vi "interface_configuration.vi"(8 "error in (no error)":errorcluster, 11 "config in":T1) -> (0 "error out":errorcluster, 3 "config out":T1)   [LabVIEW 2015, in "lv-builder-default.lvlib"]
uses:
  lv-builder-default.lvlib
  _controls/post_action_lvlib.ctl
  _controls/post_action_installer.ctl
  _controls/post_action_application.ctl
  _controls/post_action_zip.ctl
  community/_controls/configuration.ctl
  <vilib>/Utility/error.llb/Error Cluster From Error Code.vi
  <vilib>/ErrorRing/Error Ring.xnode
panel:
  in  "distribution_folder":path caption="Distribution Folder"
  in  "dependencies_folder":path caption="Dependencies Folder"
  in  "bin_folder":path caption="Bin Path"
  in  "application_post_action":T2 caption="Application Post Action"
  in  "cancel":bool
  in  "save":bool
  in  "installer_post_file":path caption="Installer Post File"
  in  "zip_move_directory":path caption="Archive Directory"
  in  "zip_post_action":T3 caption="Archive Post Action"
  in  "installer_post_action":T4 caption="Installer Post Action"
  in  "update_version_vi":path caption="Update Version VI"
  in  "lvlibp_move_directory":path caption="lvlibp Directory"
  in  "lvlib_move_directory":path caption="lvlib Directory"
  in  "lvlib_post_action":T5 caption="LVLIB Post Action"
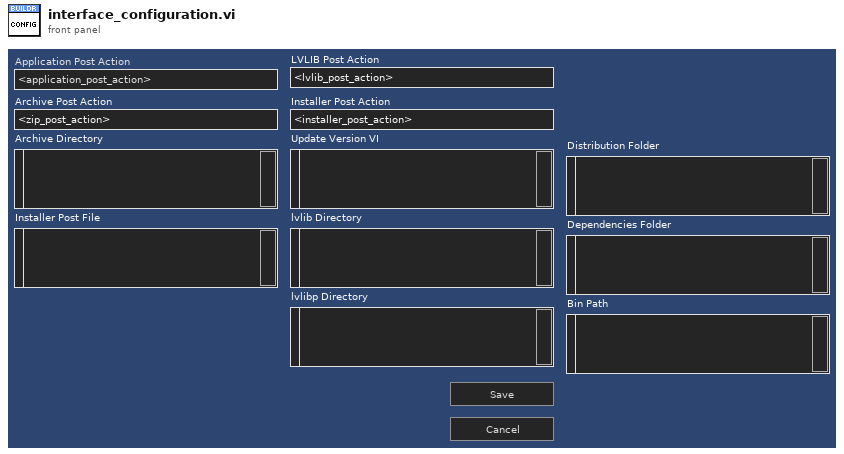
[diagram p1: front panel]
types:
  T1 = typedef "lv-builder-default.lvlib/configuration.ctl" = cluster{"project_file":string, "lvlibp_directory":string, "zip_directory":string, "lvlib_directory":string, "update_version_vi":string, "installer_post_file":string, "distribution_folder":string, "dependencies_folder":string, "version":string, "bin_folder":string, "lvlib_post_action":u16, "installer_post_action":u16, "application_post_action":u16, "zip_post_action":u16}
  T2 = typedef "lv-builder-default.lvlib/post_action_application.ctl" = enum16{"<application_post_action>", "nothing", "zip_application", "<null>"}
  T3 = typedef "lv-builder-default.lvlib/post_action_zip.ctl" = enum16{"<zip_post_action>", "nothing", "move", "extract", "<null>"}
  T4 = typedef "lv-builder-default.lvlib/post_action_installer.ctl" = enum16{"<installer_post_action>", "nothing", "create_installer", "zip_installer", "create_installer_file", "<null>"}
  T5 = typedef "lv-builder-default.lvlib/post_action_lvlib.ctl" = enum16{"<lvlib_post_action>", "nothing", "move", "install", "<null>"}
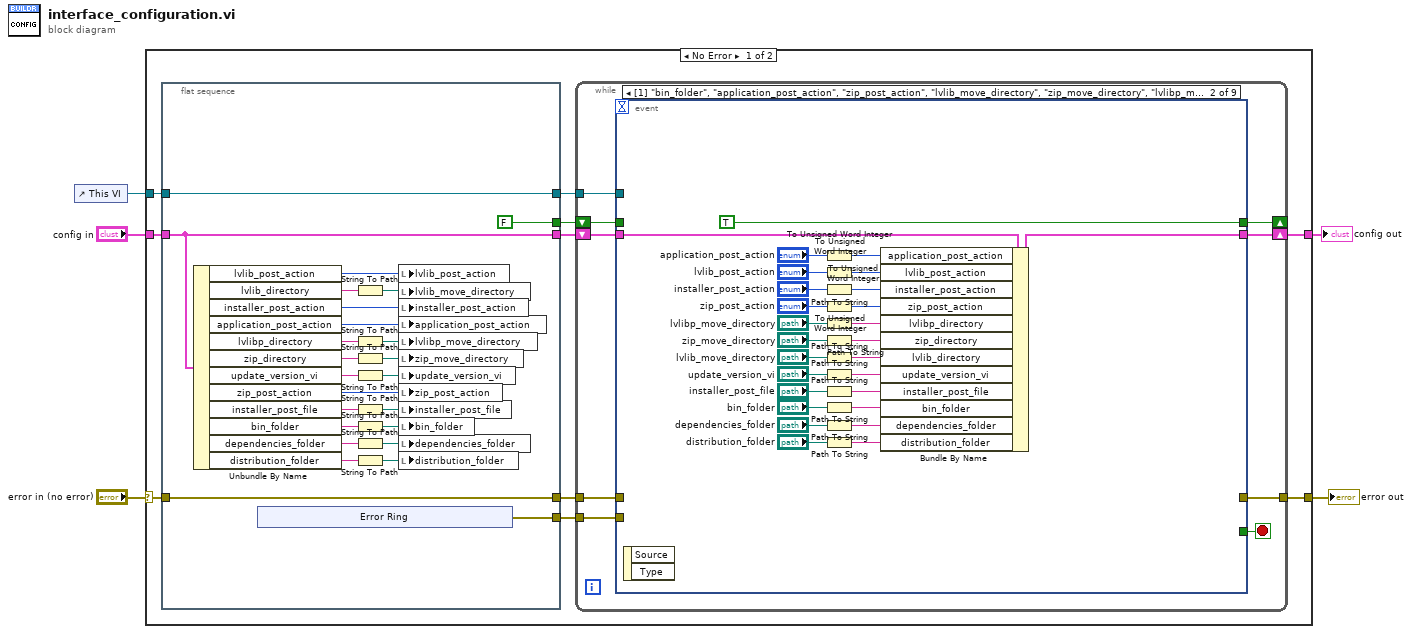
[diagram p0: block diagram]
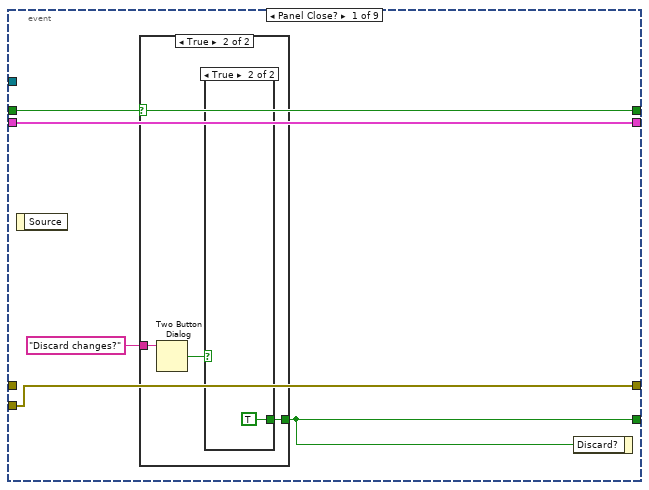
[diagram p2: hidden frame]
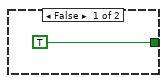
[diagram p3: hidden frame]
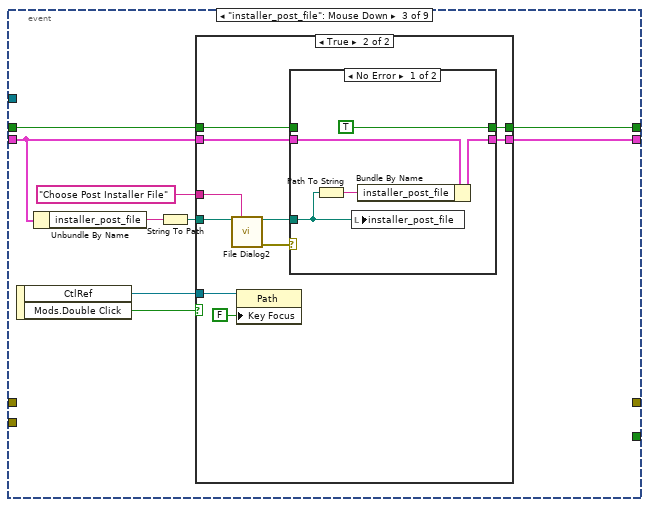
[diagram p5: hidden frame]
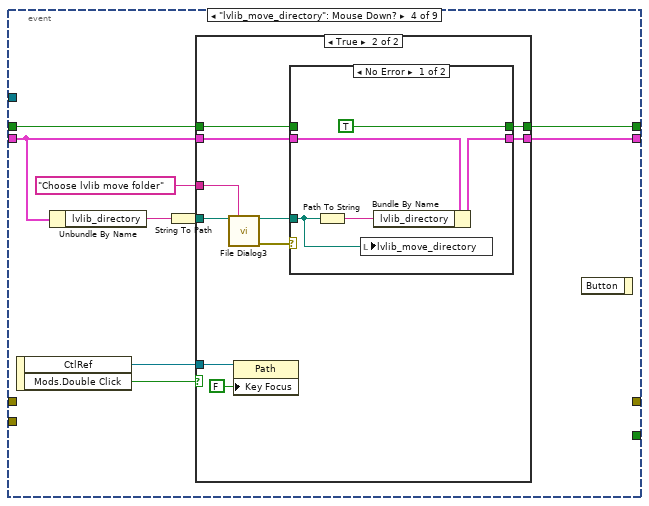
[diagram p8: hidden frame]
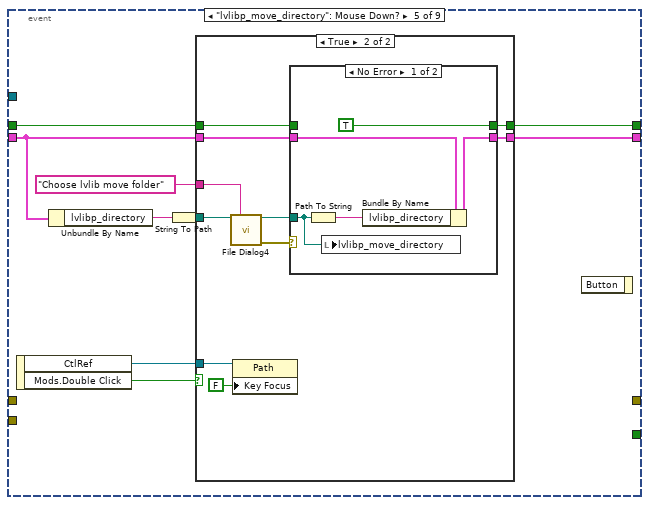
[diagram p11: hidden frame]
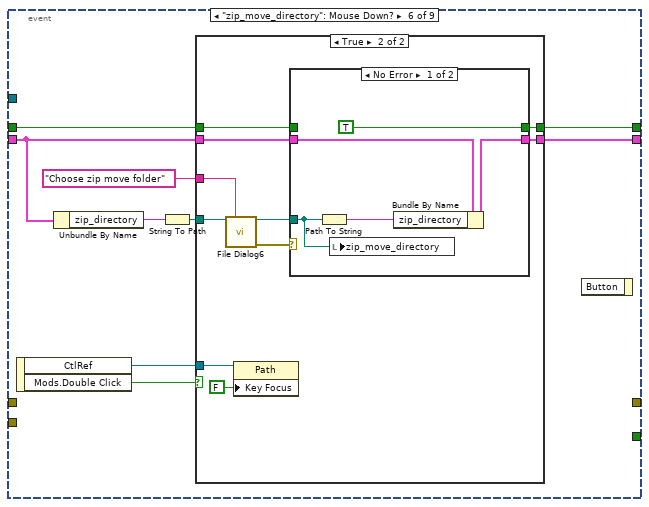
[diagram p14: hidden frame]
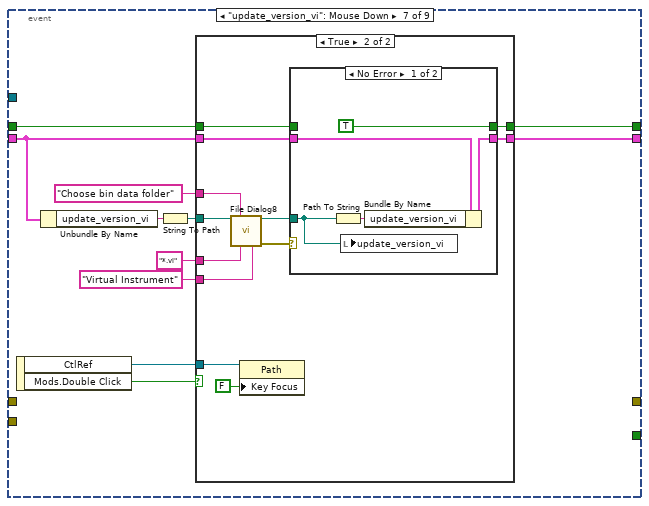
[diagram p17: hidden frame]
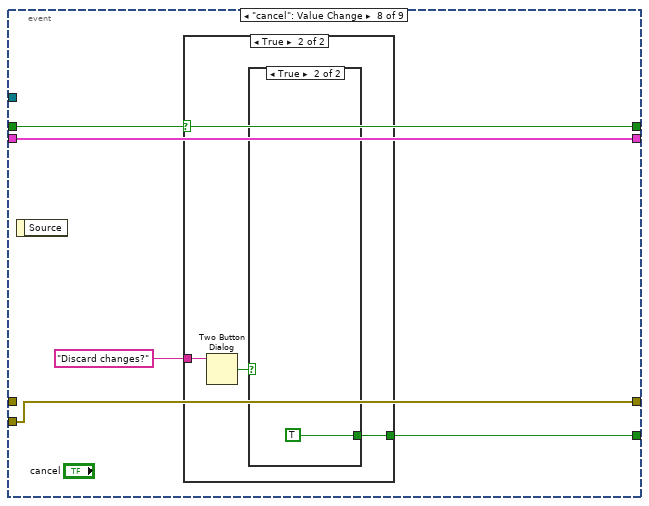
[diagram p20: hidden frame]
diagram:
  n1 = control-ref of="This VI"() -> (w3:refnum<vi>)
  n2 = case shown="No Error" "error in (no error)" {
    selector: "error in (no error)" -> [w15 w249]
    tunnel: [w9 w249] -> w4
    tunnel: w3 -> [w11 _]
    tunnel: [w8 _] -> w2
    tunnel: "config in" -> [w7 _]
    frame No Error {
      n3 = flat-sequence {
        tunnel: w15 -> [w23]
        tunnel: [w23] -> w14
        tunnel: [w24] -> w13
        tunnel: [w33] -> w12
        tunnel: w11 -> [w33]
        tunnel: [FALSE] -> w10
        tunnel: w7 -> [w24]
        tunnel: [w22] -> w6
        frame #0 {
          n4 = Unbundle By Name(w24) -> ("lvlib_post_action"=w34:u16, "lvlib_directory"=w39:string, "installer_post_action"=w35:u16, "application_post_action"=w36:u16, "lvlibp_directory"=w38:string, "zip_directory"=w37:string, "update_version_vi"=w32:string, "zip_post_action"=w31:u16, "installer_post_file"=w30:string, "bin_folder"=w21:string, "dependencies_folder"=w20:string, "distribution_folder"=w19:string)
          n5 = xnode "Error Ring"() -> ("error out"=w22:errorcluster)
          n6 = String To Path(string=w39) -> (path=w29:path)
          n7 = String To Path(string=w38) -> (path=w28:path)
          n8 = String To Path(string=w37) -> (path=w27:path)
          n9 = String To Path(string=w32) -> (path=w26:path)
          n10 = String To Path(string=w30) -> (path=w25:path)
          n11 = String To Path(string=w21) -> (path=w18:path)
          n12 = String To Path(string=w20) -> (path=w17:path)
          n13 = String To Path(string=w19) -> (path=w16:path)
          n14 = local write "lvlib_post_action"(w34) -> ()
          n15 = local write "lvlib_move_directory"(w29) -> ()
          n16 = local write "installer_post_action"(w35) -> ()
          n17 = local write "application_post_action"(w36) -> ()
          n18 = local write "lvlibp_move_directory"(w28) -> ()
          n19 = local write "zip_move_directory"(w27) -> ()
          n20 = local write "update_version_vi"(w26) -> ()
          n21 = local write "zip_post_action"(w31) -> ()
          n22 = local write "installer_post_file"(w25) -> ()
          n23 = local write "bin_folder"(w18) -> ()
          n24 = local write "dependencies_folder"(w17) -> ()
          n25 = local write "distribution_folder"(w16) -> ()
        }
      }
      n26 = while {
        tunnel: w14 -> [w46]
        shift-right: [w51] -> w8
        shift-left: w13 -> [w52]
        tunnel: w12 -> [w48]
        shift-right: [w49] -> _
        shift-left: w10 -> [w50]
        tunnel: [w47] -> w9
        tunnel: w6 -> [w45]
        stop <- w53 stop-if-true
        n27 = event shown="[1] \"bin_folder\", \"application_post_action\", \"zip_post_action\", \"lvlib_move_directory\", \"zip_move_directory\", \"lvlibp_move_directory\", \"update_version_vi\", \"installer_post_file\", \"installer_post_action\", \"dependencies_folder\", \"distribution_folder\": Value Change" {
          selector: _ -> [_ _ _ _ _ _ _ _ _]
          dyn-events: _ -> [_ _ _ _ _ _ _ _ _]
          timeout: _ -> [_ _ _ _ _ _ _ _ _]
          tunnel: [w56 _ _ _ _ _ _ w239 TRUE ("Discard?")] -> w53
          tunnel: w48 -> [_ _ _ _ _ _ _ _ _]
          tunnel: w52 -> [w58 w90 w95 w123 w151 w179 w209 w238 w247]
          tunnel: [w58 w88 w97 w125 w153 w181 w211 w238 w247] -> w51
          tunnel: w50 -> [w55 _ w99 w127 w155 w183 w213 w236 w248]
          tunnel: [w55 TRUE w98 w126 w154 w182 w212 w236 w248] -> w49
          tunnel: [w54 _ _ _ _ _ _ w235 w246] -> w47
          tunnel: w46 -> [_ _ _ _ _ _ _ _ w246]
          tunnel: w45 -> [w54 _ _ _ _ _ _ w235 _]
          event Panel Close? {
            n28 = event-data() -> ()  [unwired: 1 in, 1 out]
            n29 = case shown="True" w55 {
              tunnel: [TRUE ("Discard?") w62] -> w56
              tunnel: "Discard changes?" ("dialog_text") -> [_ w61]
              frame False {
              }
              frame True {
                n30 = Two Button Dialog(message=w61) -> (T button?=w60:bool)  [unwired: 2 in]
                n31 = case shown="True" w60 {
                  tunnel: [_ TRUE ("Discard?")] -> w62
                  frame False {
                  }
                  frame True {
                  }
                }
              }
            }
            n32 = event-data("Discard?"=w56) -> ()  [unwired: 1 in, 1 out]
          }
          event "bin_folder", "lvlib_move_directory", "zip_move_directory", "lvlibp_move_directory", "update_version_vi", "installer_post_file", "dependencies_folder", "distribution_folder": Value Change {
            n33 = event-data() -> ()  [unwired: 1 in, 2 out]
            n34 = To Unsigned Word Integer(number="application_post_action") -> (unsigned 16bit integer=w73:u16)
            n35 = To Unsigned Word Integer(number="lvlib_post_action") -> (unsigned 16bit integer=w72:u16)
            n36 = To Unsigned Word Integer(number="installer_post_action") -> (unsigned 16bit integer=w71:u16)
            n37 = To Unsigned Word Integer(number="zip_post_action") -> (unsigned 16bit integer=w70:u16)
            n38 = Path To String(path="lvlibp_move_directory") -> (string=w78:string)
            n39 = Path To String(path="zip_move_directory") -> (string=w77:string)
            n40 = Path To String(path="lvlib_move_directory") -> (string=w76:string)
            n41 = Path To String(path="update_version_vi") -> (string=w75:string)
            n42 = Path To String(path="installer_post_file") -> (string=w74:string)
            n43 = Path To String(path="bin_folder") -> (string=w64:string)
            n44 = Path To String(path="dependencies_folder") -> (string=w65:string)
            n45 = Path To String(path="distribution_folder") -> (string=w66:string)
            n46 = Bundle By Name(cluster=w90, "application_post_action"=w73, "lvlib_post_action"=w72, "installer_post_action"=w71, "zip_post_action"=w70, "lvlibp_directory"=w78, "zip_directory"=w77, "lvlib_directory"=w76, "update_version_vi"=w75, "installer_post_file"=w74, "bin_folder"=w64, "dependencies_folder"=w65, "distribution_folder"=w66) -> (w88:T1)
          }
          event "installer_post_file": Mouse Down {
            n47 = event-data() -> ("CtlRef"=w91:refnum<vi>, "Mods.Double Click"=w96:bool)  [unwired: 1 in]
            n48 = Unbundle By Name(w95) -> ("installer_post_file"=w94:string)
            n49 = String To Path(string=w94) -> (path=w92:path)
            n50 = case shown="True" w96 {
              tunnel: w99 -> [w101 w111]
              tunnel: w95 -> [w100 w110]
              tunnel: [w101 w109] -> w98
              tunnel: [w100 w108] -> w97
              tunnel: w92 -> [_ w107]
              tunnel: "Choose Post Installer File" ("description") -> [_ w106]
              tunnel: w91 -> [_ w103]
              frame False {
              }
              frame True {
                n51 = call "File Dialog2"("start path"=w107, "prompt"=w106) -> ("selected path"=w105:path, "error out"=w104:errorcluster)  [unwired: 10 in, 2 out]
                n52 = property class="Path"(reference=w103, "Key Focus"=FALSE) -> ()  [unwired: 1 in, 2 out]
                n53 = case shown="No Error" w104 {
                  tunnel: w111 -> [_ w118]
                  tunnel: w110 -> [w115 w117]
                  tunnel: [TRUE w118] -> w109
                  tunnel: [w114 w117] -> w108
                  tunnel: w105 -> [w112 _]
                  frame No Error {
                    n54 = Path To String(path=w112) -> (string=w113:string)
                    n55 = local write "installer_post_file"(w112) -> ()
                    n56 = Bundle By Name(cluster=w115, "installer_post_file"=w113) -> (w114:T1)
                  }
                  frame Error {
                  }
                }
              }
            }
          }
          event "lvlib_move_directory": Mouse Down? {
            n57 = event-data() -> ("CtlRef"=w119:refnum<vi>, "Mods.Double Click"=w124:bool)  [unwired: 1 in]
            n58 = Unbundle By Name(w123) -> ("lvlib_directory"=w122:string)
            n59 = String To Path(string=w122) -> (path=w120:path)
            n60 = case shown="True" w124 {
              tunnel: w127 -> [w129 w139]
              tunnel: w123 -> [w128 w138]
              tunnel: [w129 w137] -> w126
              tunnel: [w128 w136] -> w125
              tunnel: w120 -> [_ w134]
              tunnel: "Choose lvlib move folder" ("description") -> [_ w135]
              tunnel: w119 -> [_ w130]
              frame False {
              }
              frame True {
                n61 = call "File Dialog3"("start path"=w134, "prompt"=w135) -> ("selected path"=w133:path, "error out"=w132:errorcluster)  [unwired: 10 in, 2 out]
                n62 = property class="Path"(reference=w130, "Key Focus"=FALSE) -> ()  [unwired: 1 in, 2 out]
                n63 = case shown="No Error" w132 {
                  tunnel: w139 -> [_ w146]
                  tunnel: w138 -> [w143 w145]
                  tunnel: [TRUE w146] -> w137
                  tunnel: [w142 w145] -> w136
                  tunnel: w133 -> [w141 _]
                  frame No Error {
                    n64 = Path To String(path=w141) -> (string=w140:string)
                    n65 = local write "lvlib_move_directory"(w141) -> ()
                    n66 = Bundle By Name(cluster=w143, "lvlib_directory"=w140) -> (w142:T1)
                  }
                  frame Error {
                  }
                }
              }
            }
            n67 = event-data() -> ()  [unwired: 2 in, 1 out]
          }
          event "lvlibp_move_directory": Mouse Down? {
            n68 = event-data() -> ("CtlRef"=w147:refnum<vi>, "Mods.Double Click"=w152:bool)  [unwired: 1 in]
            n69 = Unbundle By Name(w151) -> ("lvlibp_directory"=w150:string)
            n70 = String To Path(string=w150) -> (path=w148:path)
            n71 = case shown="True" w152 {
              tunnel: w155 -> [w157 w167]
              tunnel: w151 -> [w156 w166]
              tunnel: [w157 w165] -> w154
              tunnel: [w156 w164] -> w153
              tunnel: w148 -> [_ w162]
              tunnel: "Choose lvlib move folder" ("description") -> [_ w160]
              tunnel: w147 -> [_ w158]
              frame False {
              }
              frame True {
                n72 = call "File Dialog4"("start path"=w162, "prompt"=w160) -> ("selected path"=w161:path, "error out"=w163:errorcluster)  [unwired: 10 in, 2 out]
                n73 = property class="Path"(reference=w158, "Key Focus"=FALSE) -> ()  [unwired: 1 in, 2 out]
                n74 = case shown="No Error" w163 {
                  tunnel: w167 -> [_ w174]
                  tunnel: w166 -> [w171 w173]
                  tunnel: [TRUE w174] -> w165
                  tunnel: [w170 w173] -> w164
                  tunnel: w161 -> [w169 _]
                  frame No Error {
                    n75 = Path To String(path=w169) -> (string=w168:string)
                    n76 = local write "lvlibp_move_directory"(w169) -> ()
                    n77 = Bundle By Name(cluster=w171, "lvlibp_directory"=w168) -> (w170:T1)
                  }
                  frame Error {
                  }
                }
              }
            }
            n78 = event-data() -> ()  [unwired: 2 in, 1 out]
          }
          event "zip_move_directory": Mouse Down? {
            n79 = event-data() -> ("CtlRef"=w175:refnum<vi>, "Mods.Double Click"=w180:bool)  [unwired: 1 in]
            n80 = Unbundle By Name(w179) -> ("zip_directory"=w178:string)
            n81 = String To Path(string=w178) -> (path=w176:path)
            n82 = case shown="True" w180 {
              tunnel: w183 -> [w185 w195]
              tunnel: w179 -> [w184 w194]
              tunnel: [w185 w193] -> w182
              tunnel: [w184 w192] -> w181
              tunnel: w176 -> [_ w190]
              tunnel: "Choose zip move folder" ("description") -> [_ w189]
              tunnel: w175 -> [_ w186]
              frame False {
              }
              frame True {
                n83 = call "File Dialog6"("start path"=w190, "prompt"=w189) -> ("selected path"=w191:path, "error out"=w188:errorcluster)  [unwired: 10 in, 2 out]
                n84 = property class="Path"(reference=w186, "Key Focus"=FALSE) -> ()  [unwired: 1 in, 2 out]
                n85 = case shown="No Error" w188 {
                  tunnel: w195 -> [_ w202]
                  tunnel: w194 -> [w199 w201]
                  tunnel: [TRUE w202] -> w193
                  tunnel: [w198 w201] -> w192
                  tunnel: w191 -> [w197 _]
                  frame No Error {
                    n86 = Path To String(path=w197) -> (string=w196:string)
                    n87 = local write "zip_move_directory"(w197) -> ()
                    n88 = Bundle By Name(cluster=w199, "zip_directory"=w196) -> (w198:T1)
                  }
                  frame Error {
                  }
                }
              }
            }
            n89 = event-data() -> ()  [unwired: 2 in, 1 out]
          }
          event "update_version_vi": Mouse Down {
            n90 = event-data() -> ("CtlRef"=w203:refnum<vi>, "Mods.Double Click"=w210:bool)  [unwired: 1 in]
            n91 = Unbundle By Name(w209) -> ("update_version_vi"=w208:string)
            n92 = String To Path(string=w208) -> (path=w206:path)
            n93 = case shown="True" w210 {
              tunnel: w213 -> [w215 w227]
              tunnel: w209 -> [w214 w226]
              tunnel: [w215 w225] -> w212
              tunnel: [w214 w224] -> w211
              tunnel: w206 -> [_ w223]
              tunnel: "Choose bin data folder" ("description") -> [_ w220]
              tunnel: "*.vi" ("filter") -> [_ w219]
              tunnel: "Virtual Instrument" ("filter") -> [_ w218]
              tunnel: w203 -> [_ w216]
              frame False {
              }
              frame True {
                n94 = call "File Dialog8"("start path"=w223, "prompt"=w220, "pattern (all files)"=w219, "pattern label"=w218) -> ("selected path"=w222:path, "error out"=w221:errorcluster)  [unwired: 8 in, 2 out]
                n95 = property class="Path"(reference=w216, "Key Focus"=FALSE) -> ()  [unwired: 1 in, 2 out]
                n96 = case shown="No Error" w221 {
                  tunnel: w227 -> [_ w234]
                  tunnel: w226 -> [w231 w233]
                  tunnel: [TRUE w234] -> w225
                  tunnel: [w230 w233] -> w224
                  tunnel: w222 -> [w229 _]
                  frame No Error {
                    n97 = Path To String(path=w229) -> (string=w228:string)
                    n98 = local write "update_version_vi"(w229) -> ()
                    n99 = Bundle By Name(cluster=w231, "update_version_vi"=w228) -> (w230:T1)
                  }
                  frame Error {
                  }
                }
              }
            }
          }
          event "cancel": Value Change {
            n100 = event-data() -> ()  [unwired: 1 in, 1 out]
            n101 = case shown="True" w236 {
              tunnel: [TRUE ("Discard?") w243] -> w239
              tunnel: "Discard changes?" ("dialog_text") -> [_ w241]
              frame False {
              }
              frame True {
                n102 = Two Button Dialog(message=w241) -> (T button?=w242:bool)  [unwired: 2 in]
                n103 = case shown="True" w242 {
                  tunnel: [_ TRUE ("Discard?")] -> w243
                  frame False {
                  }
                  frame True {
                  }
                }
              }
            }
          }
          event "save": Value Change {
            n104 = event-data() -> ()  [unwired: 1 in, 1 out]
          }
        }
      }
    }
    frame Error {
    }
  }
  "error out" <- w4
  "config out" <- w2
